vi "Periodic Tasks.vi"(8 "error in":errorcluster) -> ()   [LabVIEW 2016]
doc: "This VI runs in parallel to other tasks. It can contain as many user-defined periodic loops as you need. These can carry out PID or other sorts of timed response."
uses:
  <vilib>/Rock Robotics/WPI/Utilities/WPI_GetSetVariantRefNum.vi
  <vilib>/Instr/_visa.llb/VISA Configure Serial Port (Instr).vi
panel:
  out "I2C Out":u8[](array[numeric])
  in  "input string":string
  out "Positions":i32[](array[numeric])
  out "Data Out 3":u8[](array[numeric])
  in  "Numeric":i32
  out "read buffer":string
  in  "Search_Params":string[](array[string])=["x1", "y1", "z1", "x2", "y2", "z2"]
  out "Last Complete Message":string
  out "length":i32
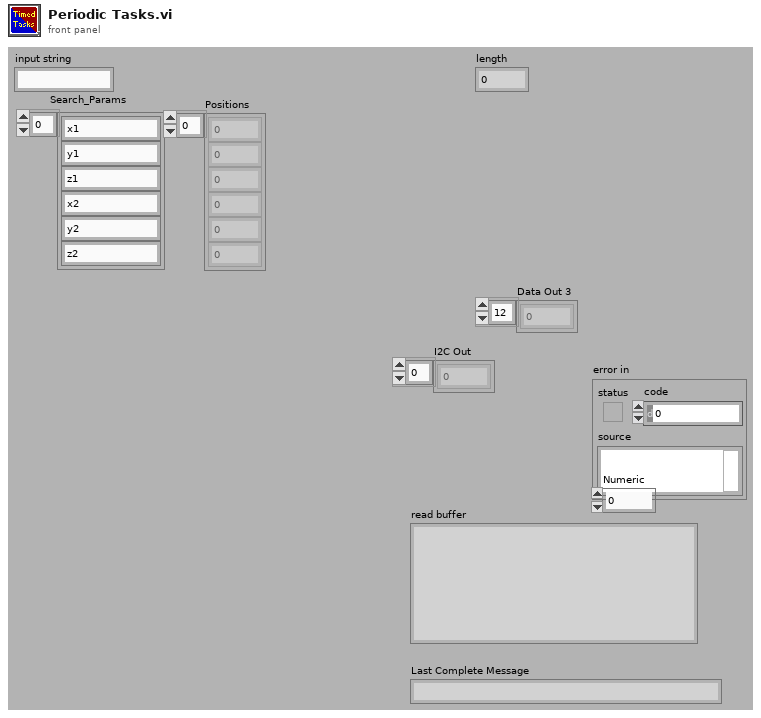
[diagram p1: front panel]
types:
  T1 = typedef "WPI_SPIDevRef.ctl" = cluster{"DevStatus":errorcluster, "Handle":i32, "SPI Bus":T2}
  T2 = typedef "spi_bus.ctl" = enum16{"SPI On-Board, CS0", "SPI On-Board, CS1", "SPI On-Board, CS2", "SPI On-Board, CS3", "SPI MXP", "Invalid"}
  T3 = typedef "WPI_I2CDevRef.ctl" = cluster{"DevStatus":errorcluster, "Device Address":u8, "Handle":i32, "I2C Bus":T4}
  T4 = typedef "i2c_bus.ctl" = enum16{"I2C On-Board", "I2C MXP", "Invalid"}
  T5 = typedef "WPI_JoystickDevRef.ctl" = cluster{"Device":T6}
  T6 = typedef "WPI_JoystickDeviceEnum.ctl" = enum16{"USB 0", "USB 1", "USB 2", "USB 3", "USB 4", "USB 5"}
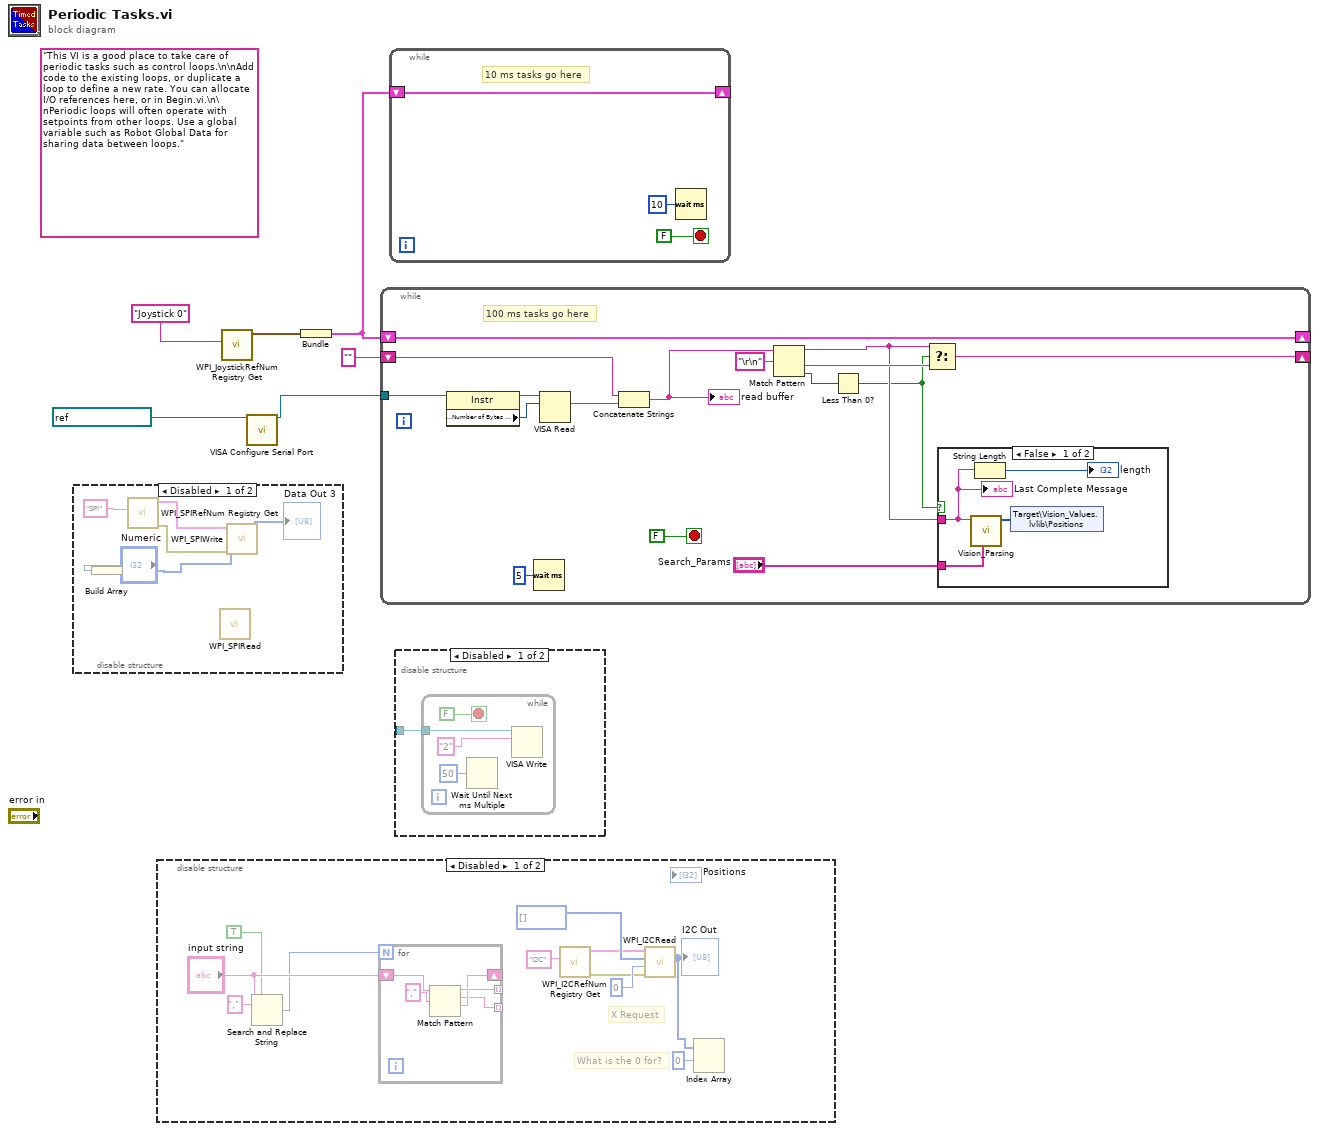
[diagram p0: block diagram]
diagram:
  (unwired) "This VI is a good place to take care of periodic tasks such as control loops.\n\nAdd code to the existing loops, or duplicate a loop to define a new rate. You can allocate I/O references here, or in Begin.vi.\n\nPeriodic loops will often operate with setpoints from other loops. Use a global variable such as Robot Global Data for sharing data between loops."
  n1 = disable-structure shown="Disabled" {
    frame Disabled {
      n2 = Build Array("Numeric") -> (w8:i32[])
      n3 = call <vilib>:"WPI_SPIRefNum Registry Get.vi"("refnum name"="SPI") -> ("error out"=w10:errorcluster, "SPIDevRef"=w11:T1)  [unwired: 9 in]
      n4 = call <vilib>:"WPI_SPIRead.vi"() -> ()  [unwired: 9 in, 3 out]
      n5 = call <vilib>:"WPI_SPIWrite.vi"("error in (no error)"=w10, "Data To Send"=w8, "SPIDevRef"=w11) -> ("Received Data"=→"Data Out 3":u8[])  [unwired: 6 in, 2 out]
    }
    frame Enabled {
    }
  }
  n6 = disable-structure shown="Disabled" {
    frame Disabled {
      # "What is the 0 for?"
      # "X Request"
      n7 = Search and Replace String(replace all?=TRUE ("replace all? (F)"), input string="input string", search string=",") -> (number of replacements=w14:i32)  [unwired: 5 in, 3 out]
      n8 = for {
        N: w14 -> [_]
        tunnel: [w27] -> _ mode=indexing
        shift-right: [w25] -> _
        shift-left: "input string" -> [w26]
        tunnel: [w24] -> _ mode=indexing
        n9 = Match Pattern(string=w26, regular expression=",") -> (before substring=w27:string, match substring=w24:string, after substring=w25:string)  [unwired: 1 in, 1 out]
      }
      n10 = call <vilib>:"WPI_I2CRefNum Registry Get.vi"("refnum name"="I2C") -> ("error out"=w17:errorcluster, "I2CDevRef"=w18:T3)  [unwired: 9 in]
      n11 = call <vilib>:"WPI_I2CRead.vi"("error in (no error)"=w17, "I2CBytesToRead"=u8 0, "I2CRegister"=u8[] [], "I2CDevRef"=w18) -> ("Data Out"=w20:u8[])  [unwired: 5 in, 2 out]
      "I2C Out" <- w20
      n12 = Index Array(array=w20, index #1=0 ("index")) -> ()  [unwired: 1 in, 2 out]
    }
    frame Enabled {
    }
  }
  n13 = call <vilib>:"WPI_JoystickRefNum Registry Get.vi"("refnum name"="Joystick 0") -> ("JoystickDevRef"=w5:T5)  [unwired: 1 in, 9 out]
  n14 = call-poly "VISA Configure Serial Port"("VISA resource name"=refnum<visa-resource-name> "ASRL2::INSTR") -> ("VISA resource name out"=w2:refnum<visa-resource-name>)  [unwired: 13 in, 1 out]
  n15 = Bundle("JoystickDevRef"=w5) -> (w4:cluster{"JoystickDevRef":T5})  [unwired: 1 out]
  n16 = while {
    shift-right: [w43] -> _
    shift-left: w4 -> [w43]
    tunnel: w2 -> [w38]
    shift-right: [w30] -> _
    shift-left: "" -> [w37]
    stop <- FALSE stop-if-true
    # "100 ms tasks go here"
    n17 = property class="Instr"(reference=w38) -> (reference out=w42:refnum<visa-resource-name>, "Serial Settings:Number of Bytes at Serial Port"=w41:u32)  [unwired: 1 in, 1 out]
    n18 = Wait (ms)(milliseconds to wait=u32 5) -> ()  [unwired: 1 out]
    n19 = VISA Read(VISA resource name=w42, byte count=w41) -> (read buffer=w36:string)  [unwired: 1 in, 3 out]
    n20 = Concatenate Strings(w37, w36) -> (w35:string)
    "read buffer" <- w35
    n21 = Match Pattern(string=w35, regular expression="\r\n") -> (before substring=w31:string, after substring=w32:string, offset past match=w33:i32)  [unwired: 1 in, 1 out]
    n22 = Less Than 0?(x=w33) -> (x < 0?=w29:bool)
    n23 = Select(t=w31, s=w29, f=w32) -> (s? t:f=w30:string)
    n24 = case shown="False" w29 {
      tunnel: "Search_Params" -> [w48 _]
      tunnel: w31 -> [w47 _]
      frame False {
        n25 = call "Vision_Parsing.vi"("Search_Params"=w48, "Input"=w47) -> ("Positions"=w45:i32[])  [unwired: 9 in]
        n26 = String Length(string=w47) -> (length=→"length":i32)
        n27 = shared-variable "Target\\Vision_Values.lvlib\\Positions"(w45) -> ()  [unwired: 1 in, 1 out]
        "Last Complete Message" <- w47
      }
      frame True {
      }
    }
  }
  n28 = while {
    shift-right: [w49] -> _
    shift-left: w4 -> [w49]
    stop <- FALSE stop-if-true
    # "10 ms tasks go here"
    n29 = Wait (ms)(milliseconds to wait=u32 10) -> ()  [unwired: 1 out]
  }
  n30 = disable-structure shown="Disabled" {
    disable-tunnel: _ -> [w52 _]
    frame Disabled {
      n31 = while {
        tunnel: w52 -> [w55]
        stop <- FALSE stop-if-true
        n32 = Wait Until Next ms Multiple(millisecond multiple=u32 50) -> ()  [unwired: 1 out]
        n33 = VISA Write(VISA resource name=w55, write buffer="2" ("write buffer 2")) -> ()  [unwired: 1 in, 3 out]
      }
    }
    frame Enabled {
    }
  }
